vi "BLAS2 Utility(DBL).vi"(0 "x":dbl[](array[numeric]), 1 "y":dbl[](array[numeric]), 2 "A":T3, 3 "operation A":T2 items=["Direct", "Conjugated & Transposed", "Transposed"], 6 "function":T1 items=["ddot/zdotu/zdotc", "daxpy/zaxpy", "dnrm2/dznrm2", "dasum/dzasum", "dcopy/zcopy", "dswap/zswap", "drotm", "drot/zdrot", "idamax/izamax", "idamin/izamin", "dgemv/zgemv", "dsymv/zhemv", "dtrmv/ztrmv", "dsyr/zher", "dsyr2/zher2", "dger/zgeru/zgerc", "dtrsv/ztrsv", "dgemm/zgemm", "dsymm/zsymm/zhemm", "dtrmm/ztrmm", "dsyrk/zsyrk/zherk", "dsyr2k/zsyr2k/zher2k", "dtrsm/ztrsm"]) -> (13 "m":i32, 14 "lda":i32, 19 "n":i32)   [LabVIEW 2014, in "NI_AALBLAS.lvlib"]
uses:
  NI_AALBLAS.lvlib
  RealMatrix.ctl
  LV_Transpose.ctl
  Fucntion.ctl
  NI_Matrix.lvlib
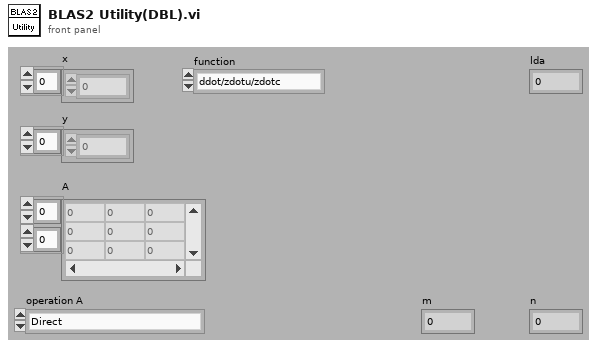
[diagram p1: front panel]
types:
  T1 = typedef "NI_AALBLAS.lvlib/Fucntion.ctl" = u16
  T2 = typedef "NI_AALBLAS.lvlib/LV_Transpose.ctl" = i32
  T3 = typedef "NI_Matrix.lvlib/RealMatrix.ctl" = dbl[][]
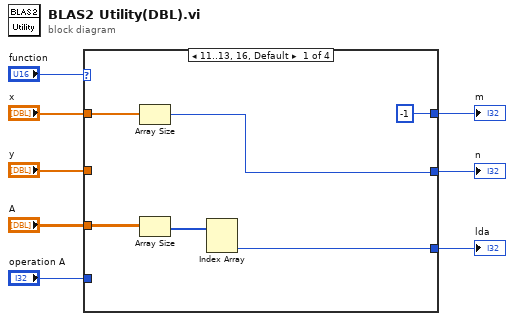
[diagram p0: block diagram]
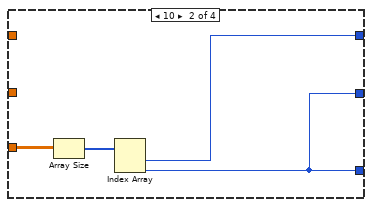
[diagram p2: hidden frame]
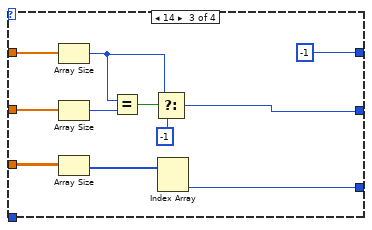
[diagram p3: hidden frame]
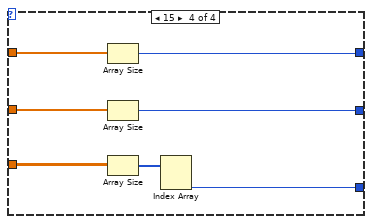
[diagram p4: hidden frame]
diagram:
  n1 = case shown="11..13, 16, Default" "function" {
    tunnel: "x" -> [w14 _ w29 w36]
    tunnel: "y" -> [_ _ w28 w34]
    tunnel: "A" -> [w11 w18 w20 w31]
    tunnel: "operation A" -> [_ _ _ _]
    tunnel: [w13 w15 w24 w32] -> w4
    tunnel: [-1 w16 -1 w35] -> w3
    tunnel: [w9 w15 w19 w30] -> w1
    frame 11..13, 16, Default {
      n2 = Array Size(array=w14) -> (size(s)=w13:i32)
      n3 = Array Size(array=w11) -> (size(s)=w10:i32[])
      n4 = Index Array(array=w10) -> (element #2=w9:i32)  [unwired: 2 in, 1 out]
    }
    frame 10 {
      n5 = Array Size(array=w18) -> (size(s)=w17:i32[])
      n6 = Index Array(array=w17) -> (element #1=w16:i32, element #2=w15:i32)  [unwired: 2 in]
    }
    frame 14 {
      n7 = Array Size(array=w29) -> (size(s)=w25:i32)
      n8 = Array Size(array=w28) -> (size(s)=w27:i32)
      n9 = Array Size(array=w20) -> (size(s)=w21:i32[])
      n10 = Equal?(x=w25, y=w27) -> (x = y?=w26:bool)
      n11 = Select(t=w25, s=w26, f=-1) -> (s? t:f=w24:i32)
      n12 = Index Array(array=w21) -> (element #2=w19:i32)  [unwired: 2 in, 1 out]
    }
    frame 15 {
      n13 = Array Size(array=w36) -> (size(s)=w35:i32)
      n14 = Array Size(array=w34) -> (size(s)=w32:i32)
      n15 = Array Size(array=w31) -> (size(s)=w33:i32[])
      n16 = Index Array(array=w33) -> (element #2=w30:i32)  [unwired: 2 in, 1 out]
    }
  }
  "n" <- w4
  "m" <- w3
  "lda" <- w1
